vi "Object.vi"() -> (3 "SceneObject out":refnum<vi>)   [LabVIEW 2022 SP3]
uses:
  <vilib>/picture/3D Picture Control/Object/Create Object (name).vi
  <vilib>/picture/3D Picture Control/NI_3D Picture Control.lvlib
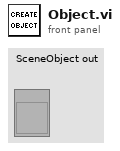
[diagram p1: front panel]
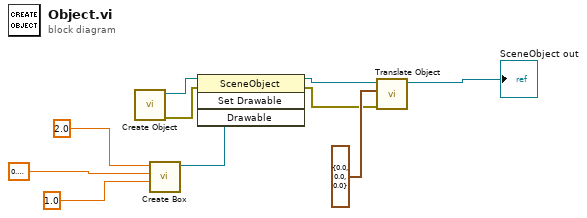
[diagram p0: block diagram]
diagram:
  n1 = call-poly <vilib>:"Create Object.vi"() -> ("error out"=w5:errorcluster, "Scene:New Object"=w4:refnum<vi>)  [unwired: 10 in]
  n2 = call <vilib>:"Create Box.vi"("Length Z"=sgl 1.0, "Length Y"=sgl 0.2, "Length X"=sgl 2.0) -> ("New Box Refnum"=w6:refnum<vi>)  [unwired: 7 in, 1 out]
  n3 = invoke class="SceneObject" method="Set Drawable"(reference=w4, error in=w5, "Drawable"=w6) -> (reference out=w7:refnum<vi>, error out=w8:errorcluster)  [unwired: 1 in, 2 out]
  n4 = call <vilib>:"Translate Object.vi"("error in (no error)"=w8, "Translation"=cluster{"X":sgl, "Y":sgl, "Z":sgl} {"X"=0.0, "Y"=0.0, "Z"=0.0}, "Scene.Object In"=w7) -> ("Scene.Object Out"=→"SceneObject out":refnum<vi>)  [unwired: 7 in, 1 out]
